vi "Load_Cell_DAQ2.vi"() -> ()   [LabVIEW 2013]
uses:
  <vilib>/Utility/error.llb/DialogType.ctl
  <vilib>/DAQmx/read.llb/DAQmx Read (Analog 2D DBL NChan NSamp).vi
  <vilib>/DAQmx/create/channels.llb/DAQmx Create Channel (AI-Voltage-Basic).vi
  <vilib>/DAQmx/configure/timing.llb/DAQmx Timing (Sample Clock).vi
  <vilib>/DAQmx/miscellaneous.llb/DAQmx Fill In Error Info.vi
  <vilib>/Utility/file.llb/Write To Spreadsheet File (DBL).vi
panel:
  out "Winner":bool
  in  "OK Button":bool
  in  "Radio Buttons":enum32{"Robot", "Human"}(radio)
  out "Robot":dbl(slide) scale=0.0..100.0
  out "Human":dbl(slide) scale=0.0..100.0
  out "Pound-Force:":dbl format="%#.2f"
  out "Newton:":dbl format="%#.2f"
  in  "Data File":path
  in  "Collect Data":bool=TRUE
  out "Voltages":dbl[][](array[numeric])
  in  "input terminal configuration":i32(ring)=10083 items=["default"=-1, "RSE"=10083, "NRSE"=10078, "Differential"=10106, "Pseudodifferential"=12529]
  out "Measurement":dbl[][](graph) caption="Load Cell Data"
  in  "stop":bool
  in  "Samples to Read":i32=100
  in  "Maximum Value":dbl=10.0 format="%0.2f"
  in  "Minimum Value":dbl=-10.0 format="%0.2f"
  in  "Sample Rate":dbl=1000.0 caption="Sample Rate (Hz)" format="%0.2f"
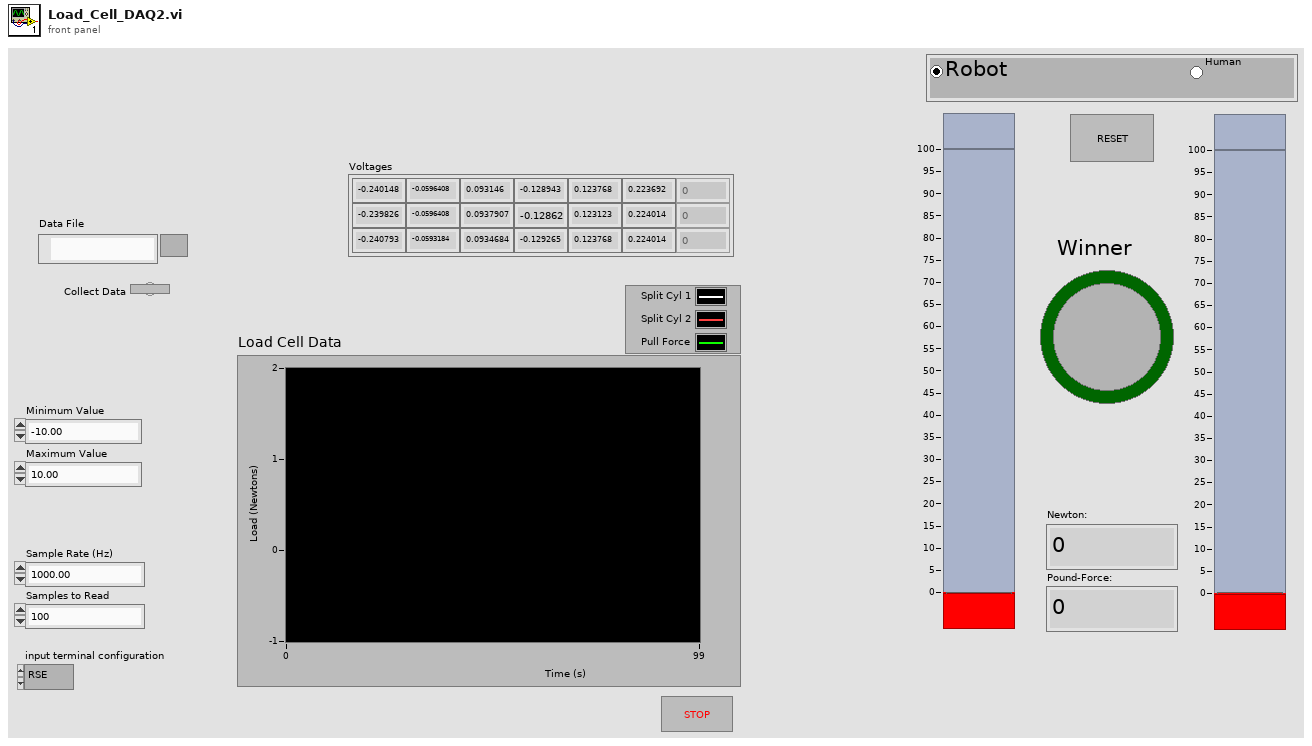
[diagram p1: front panel]
types:
  T1 = typedef "DialogType.ctl" = u16
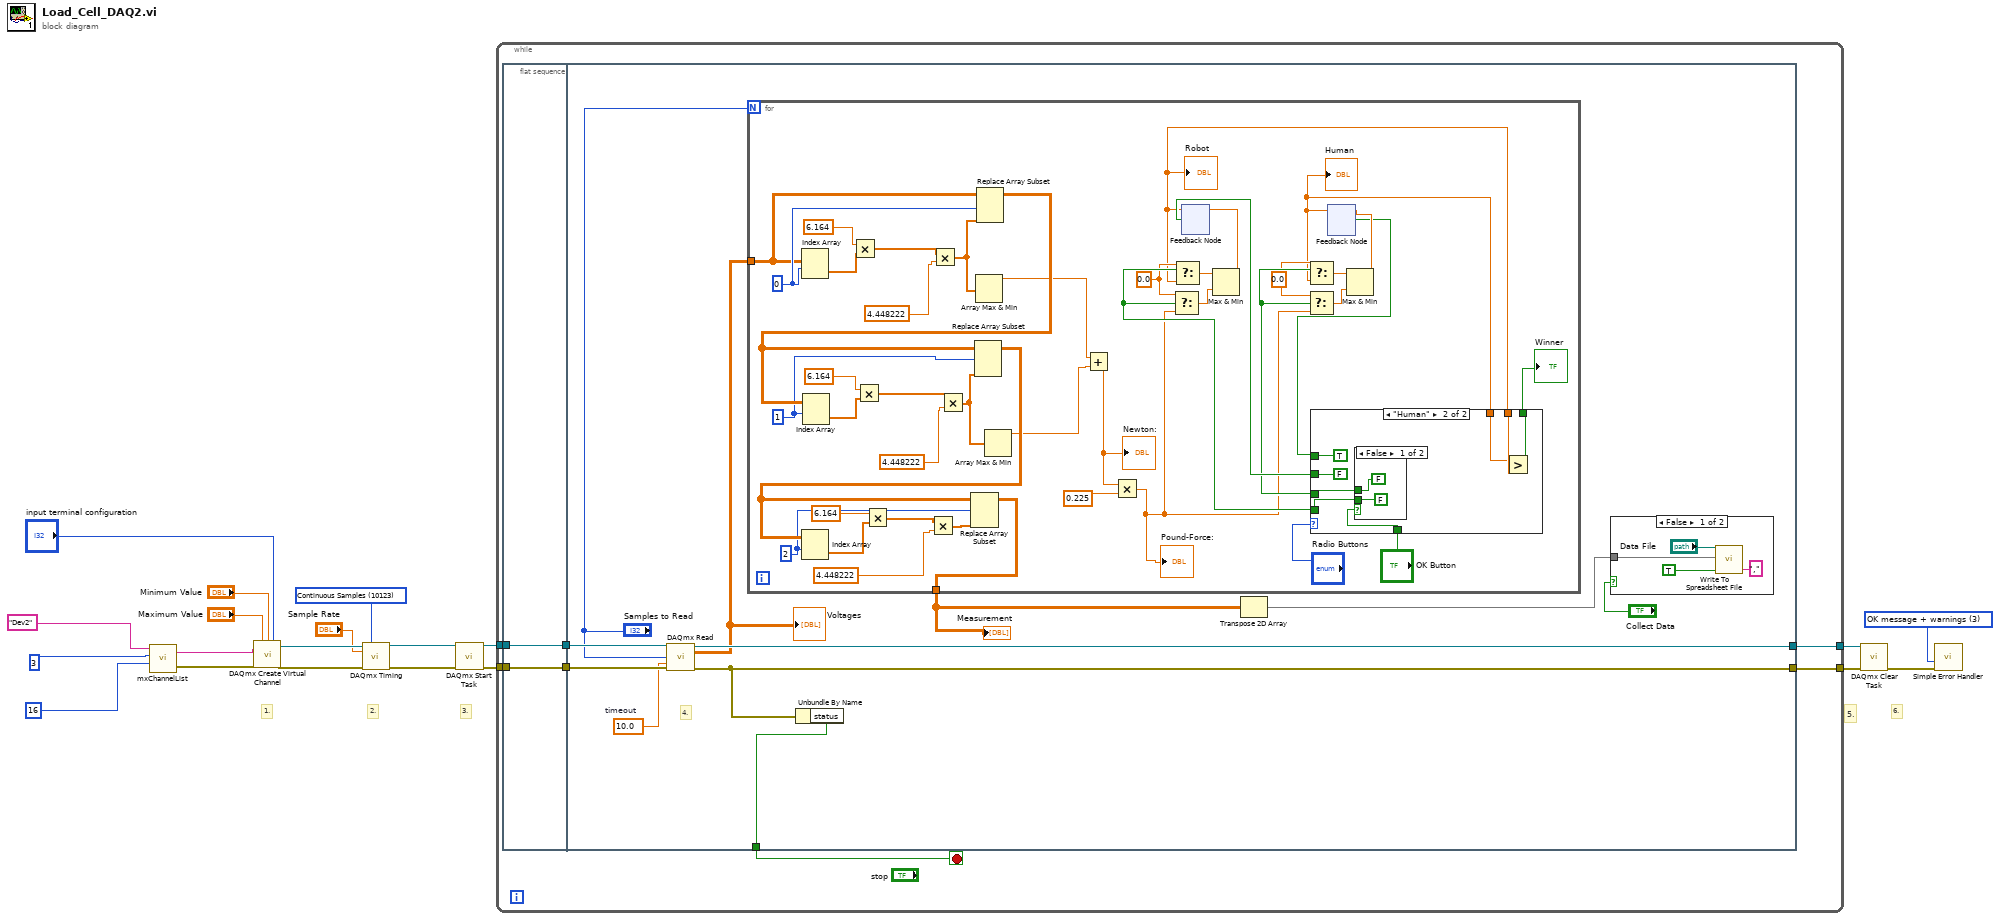
[diagram p0: block diagram]
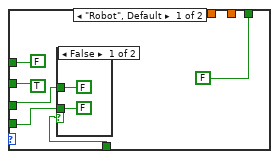
[diagram p3: hidden frame]
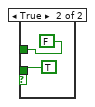
[diagram p4: hidden frame]
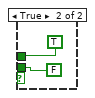
[diagram p5: hidden frame]
diagram:
  w7 = T1 3 items=["no dialog", "OK message", "continue or stop message", "OK message + warnings", "continue/stop + warnings"] ("type of dialog (OK msg:1)")
  w12 = 10123 items=["Finite Samples"=10178, "Continuous Samples"=10123] ("sample mode")
  # "6."
  # "5."
  # "3."
  # "2."
  # "1."
  n1 = call "mxChannelList.vi"("First Channel"=i16 16, "Number of Channels"=i16 3, "DAQmx Device Name"="Dev2") -> ("error out"=w1:errorcluster, "Channel List"=w4:string)  [unwired: 1 in]
  n2 = call-poly <vilib>:"DAQmx Create Virtual Channel.vi"("maximum value"="Maximum Value", "minimum value"="Minimum Value", "input terminal configuration"="input terminal configuration", "physical channels"=w4, "error in"=w1) -> ("task out"=w15:refnum<k21>, "error out"=w18:errorcluster)  [unwired: 9 in]
  n3 = call-poly <vilib>:"DAQmx Timing.vi"("task/channels in"=w15, "sample mode"=w12, "rate"="Sample Rate", "error in"=w18) -> ("task out"=w11:refnum<k21>, "error out"=w10:errorcluster)  [unwired: 10 in]
  n4 = call <vilib>:"DAQmx Start Task.vi"("task/channels in"=w11, "error in"=w10) -> ("task out"=w14:refnum<k21>, "error out"=w17:errorcluster)  [unwired: 12 in]
  n5 = while {
    tunnel: w17 -> [w27]
    tunnel: w14 -> [w26]
    tunnel: [w25] -> w13
    tunnel: [w24] -> w9
    stop <- w21 stop-if-true
    n6 = flat-sequence {
      tunnel: w26 -> [w28]
      tunnel: w27 -> [w29]
      tunnel: [w29] -> w23
      tunnel: [w28] -> w22
      tunnel: [w38] -> w25
      tunnel: [w37] -> w24
      tunnel: [w36] -> w21
      tunnel: w23 -> [w40]
      tunnel: w22 -> [w39]
      frame #0 {
      }
      frame #1 {
        w35 = 10.0  # timeout
        # "4."
        n7 = call-poly <vilib>:"DAQmx Read.vi"("task/channels in"=w39, "number of samples per channel"="Samples to Read", "timeout"=w35, "error in"=w40) -> ("task out"=w38:refnum<k21>, "data"=w33:dbl[][], "error out"=w37:errorcluster)  [unwired: 9 in]
        "Voltages" <- w33
        n8 = for {
          N: "Samples to Read" -> [_]
          tunnel: w33 -> [w81]
          tunnel: [w76] -> w31
          w48 = 0.0
          w50 = 0.0
          w77 = i16 2
          w79 = i16 1
          w82 = i16 0
          n9 = Index Array(array=w81, index (row)=w82) -> (element=w85:dbl[])  [unwired: 1 in]
          n10 = Multiply(x=6.164, y=w85) -> (x*y=w72:dbl[])
          n11 = Multiply(x=w72, y=4.448222) -> (x*y=w69:dbl[])
          n12 = Array Max & Min(array=w69) -> (max value=w66:dbl)  [unwired: 3 out]
          n13 = Replace Array Subset(array=w81, new element=w69, index (row)=w82) -> (w80:dbl[][])  [unwired: 1 in]
          n14 = Index Array(array=w80, index (row)=w79) -> (element=w84:dbl[])  [unwired: 1 in]
          n15 = Multiply(x=6.164, y=w84) -> (x*y=w71:dbl[])
          n16 = Multiply(x=w71, y=4.448222) -> (x*y=w67:dbl[])
          n17 = Replace Array Subset(array=w80, new element=w67, index (row)=w79) -> (w78:dbl[][])  [unwired: 1 in]
          n18 = Index Array(array=w78, index (row)=w77) -> (element=w83:dbl[])  [unwired: 1 in]
          n19 = Multiply(x=6.164, y=w83) -> (x*y=w70:dbl[])
          n20 = Multiply(x=w70, y=4.448222) -> (x*y=w68:dbl[])
          n21 = Replace Array Subset(array=w78, new element=w68, index (row)=w77) -> (w76:dbl[][])  [unwired: 1 in]
          n22 = Array Max & Min(array=w67) -> (max value=w65:dbl)  [unwired: 3 out]
          n23 = Add(x=w66, y=w65) -> (x+y=w64:dbl)
          "Newton:" <- w64
          n24 = Multiply(x=w64, y=0.225) -> (x*y=w49:dbl)
          "Pound-Force:" <- w49
          n25 = feedback #1() -> (w46:dbl)  [unwired: 1 in]
          "Robot" <- w46
          n26 = feedback #2() -> (w47:dbl)  [unwired: 1 in]
          "Human" <- w47
          n27 = case shown="\"Human\"" "Radio Buttons" {
            tunnel: [FALSE TRUE] -> w55
            tunnel: [TRUE FALSE] -> w54
            tunnel: "OK Button" -> [w92 w104]
            tunnel: [w90 w103] -> w52
            tunnel: [w91 w102] -> w51
            tunnel: w47 -> [_ w100]
            tunnel: w46 -> [_ w101]
            tunnel: [FALSE w99] -> w45
            frame "Robot", Default {
              n28 = case shown="False" w92 {
                tunnel: [FALSE TRUE] -> w91
                tunnel: [FALSE FALSE] -> w90
                frame False {
                }
                frame True {
                }
              }
            }
            frame "Human" {
              n29 = case shown="False" w104 {
                tunnel: [FALSE TRUE] -> w103
                tunnel: [FALSE FALSE] -> w102
                frame False {
                }
                frame True {
                }
              }
              n30 = Greater?(x=w100, y=w101) -> (0:w99:bool)
            }
          }
          "Winner" <- w45
          n31 = Select(t=w50, s=w51, f=w49) -> (s? t:f=w60:dbl)
          n32 = Select(t=w50, s=w51, f=w46) -> (s? t:f=w61:dbl)
          n33 = Max & Min(x=w61, y=w60) -> (max(x,y)=w62:dbl)  [unwired: 1 out]
          n34 = feedback-in #1(w62, w54) -> ()
          n35 = Select(t=w48, s=w52, f=w49) -> (s? t:f=w58:dbl)
          n36 = Select(t=w48, s=w52, f=w47) -> (s? t:f=w59:dbl)
          n37 = Max & Min(x=w59, y=w58) -> (max(x,y)=w57:dbl)  [unwired: 1 out]
          n38 = feedback-in #2(w57, w55) -> ()
        }
        "Measurement" <- w31
        n39 = Unbundle By Name(w37) -> ("status"=w36:bool)
        n40 = Transpose 2D Array(2D array=w31) -> (transposed array=w30:dbl[][])
        n41 = case shown="False" "Collect Data" {
          tunnel: w30 -> [w44 _]
          frame False {
            n42 = call-poly <vilib>:"Write To Spreadsheet File.vi"("delimiter (\\t)"=",", "append to file? (new file:F)"=TRUE, "2D data"=w44, "file path (dialog if empty)"="Data File") -> ()  [unwired: 4 in, 1 out]
          }
          frame True {
          }
        }
      }
    }
  }
  n43 = call <vilib>:"DAQmx Clear Task.vi"("task in"=w13, "error in"=w9) -> ("error out"=w16:errorcluster)  [unwired: 13 in]
  n44 = call <vilib>:"Simple Error Handler.vi"("type of dialog (OK msg:1)"=w7, "error in (no error)"=w16) -> ()  [unwired: 3 in, 5 out]
